vi "數位濾波版V2.vi"() -> ()   [LabVIEW 2010]
uses:
  <vilib>/Analysis/3filter.llb/Filter Passband Type.ctl
  <vilib>/DAQmx/read.llb/DAQmx Read (Analog DBL 1Chan 1Samp).vi
  <vilib>/DAQmx/write.llb/DAQmx Write (Analog DBL 1Chan 1Samp).vi
  <vilib>/DAQmx/create/channels.llb/DAQmx Create Channel (AI-Voltage-Basic).vi
  <vilib>/DAQmx/configure/timing.llb/DAQmx Timing (Sample Clock).vi
  <vilib>/DAQmx/create/channels.llb/DAQmx Create Channel (AO-Voltage-Basic).vi
  <vilib>/daqmx/miscellaneous.llb/DAQmx Fill In Error Info.vi
  <vilib>/Analysis/3filter.llb/Butterworth Filter (DBL).vi
  <vilib>/Analysis/NI_AALBase.lvlib
panel:
  in  "濾波?":bool
  in  "low cutoff freq: fl":dbl=200.0 format="%0.4f"
  out "理想迴圈時間":dbl
  out "延遲警告":bool
  in  "濾波階數":i32=6
  out "當下DC值":dbl
  in  "DAQ input":tag
  in  "DAQ output":tag
  in  "平均數":i32=1
  in  "ÂoDC«á©ñ¤j":dbl=1.0
  in  "Kp":dbl=1.0
  out "當下誤差":dbl=0.1 format="%#_13g"
  out "message":string=" INSTRUCTIONS:\r\rNormal Use:  When using subVIs that incorporate the error in/error out (or error I/O) structure, place this handler where you want to inform the user of an error, typically at the end of the I/O data path, as the last action of the program.  If the error in error? is ERROR, the handler creates a message describing the error and its source.  If the type of dialog = 1 (default), the message is displayed to the user, who can only acknowedge it.  If the type = 2, the user can acknowledge the message or abort execution; aborting a program with active I/O is not recommended.  If the type = 0, no message is displayed; this is used to process the error programmatically, and the error out cluster elements are wired to individual terminals for that reason.  \r\rOther Use:\n\r\nlocal testing.  To test the error code of a subVI or function that does not have the error I/O structure, you can wire its error code and a source string to the local error code and error source inputs.  If error in error? indicates no error and error code is not equal to 0, the local code and source are substituted for the error in values, and error? is set TRUE (ERROR)."
  out "while平均運行時間":dbl
  in  "取樣頻率":dbl=9000.0 min=1.0 max=20000.0 step=1.0
  in  "stop":bool
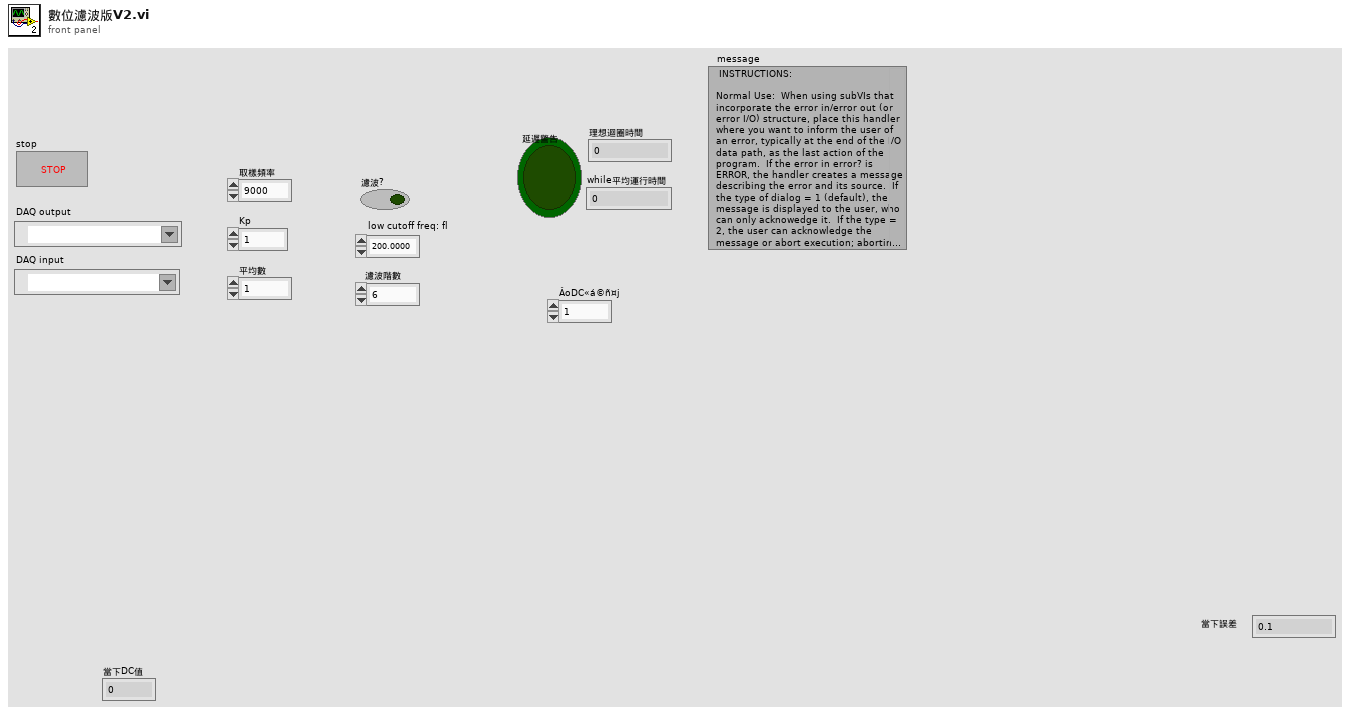
[diagram p1: front panel]
types:
  T1 = typedef "NI_AALBase.lvlib/Filter Passband Type.ctl" = enum32{"Lowpass", "Highpass", "Bandpass", "Bandstop"}
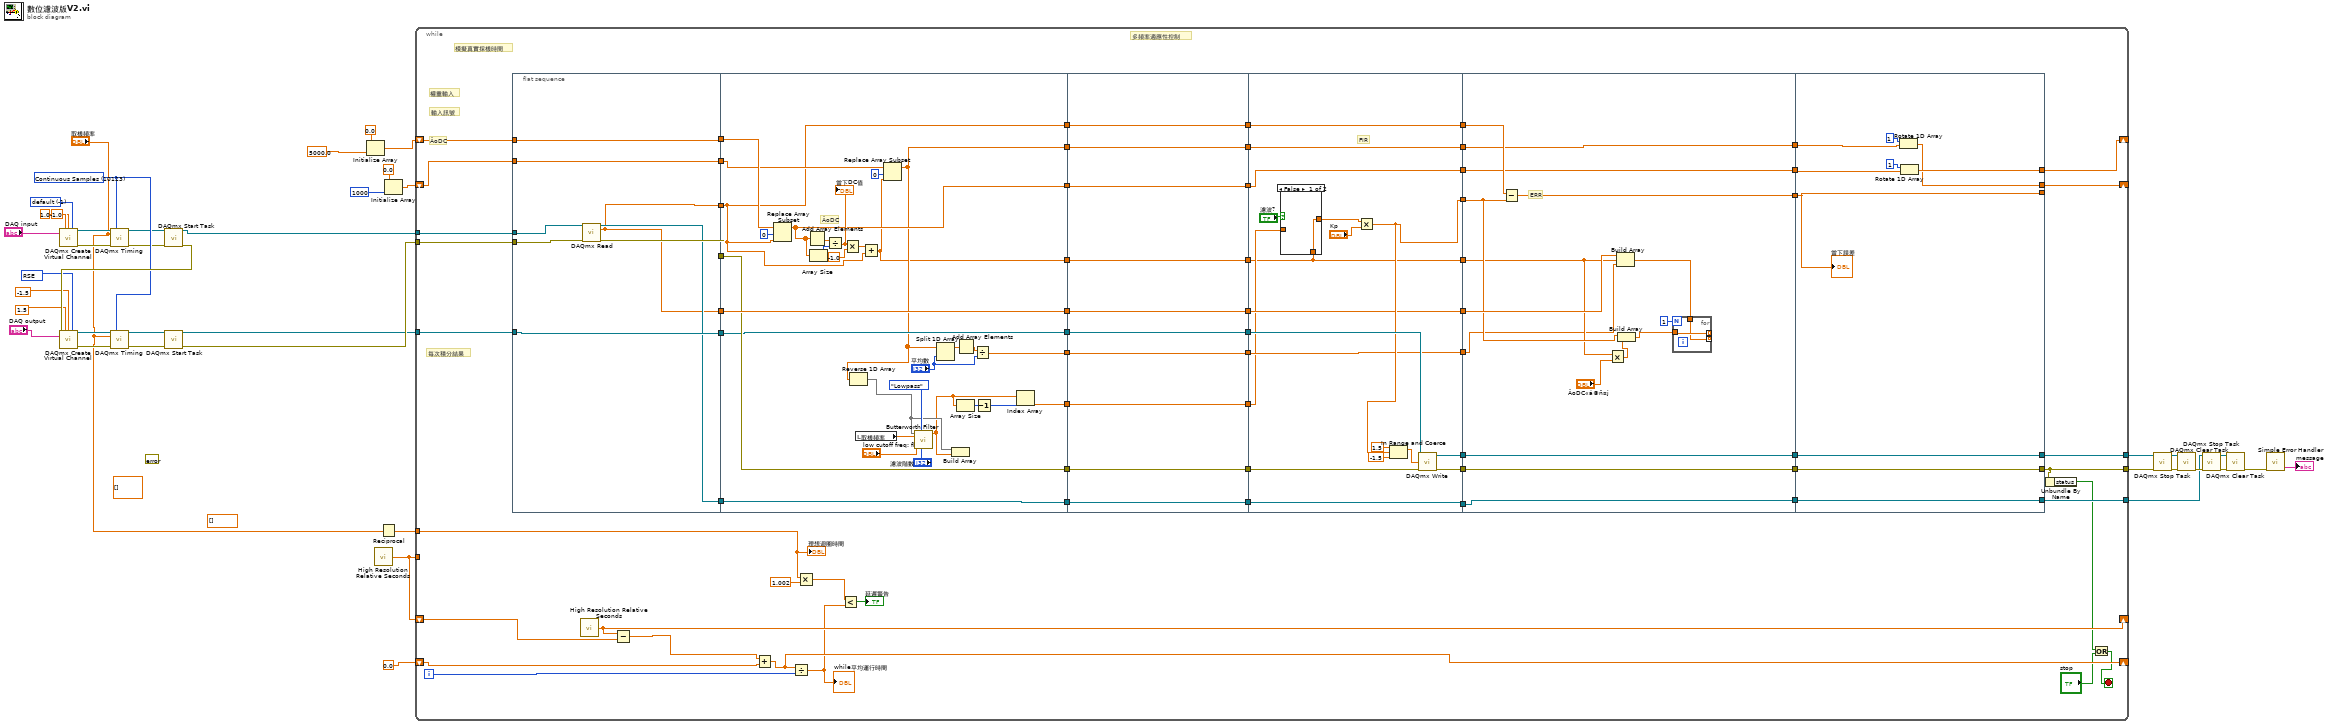
[diagram p0: block diagram]
diagram:
  w34 = 10123 items=["Finite Samples"=10178, "Continuous Samples"=10123, "Hardware Timed Single Point"=12522] ("sample mode")
  w31 = 10083 items=["Default"=-1, "RSE"=10083, "Differential"=10106, "Pseudodifferential"=12529] ("output terminal configuration")
  w30 = -1 items=["default"=-1, "RSE"=10083, "NRSE"=10078, "Differential"=10106, "Pseudodifferential"=12529] ("input terminal configuration")
  (unwired) dbl[] [] ("History Data")
  (unwired) dbl[][] [] ("History Data")
  (unwired) errorcluster {"status"=FALSE, "code"=0, "source"=""} ("error constant")
  n1 = call-poly <vilib>:"DAQmx Create Virtual Channel.vi"("maximum value"=1.0, "minimum value"=-1.0, "input terminal configuration"=w30, "physical channels"="DAQ input") -> ("task out"=w22:refnum<k21>, "error out"=w25:errorcluster)  [unwired: 10 in]
  n2 = call-poly <vilib>:"DAQmx Timing.vi"("task/channels in"=w22, "sample mode"=w34, "rate"="取樣頻率", "error in"=w25) -> ("task out"=w23:refnum<k21>, "error out"=w24:errorcluster)  [unwired: 10 in]
  n3 = call <vilib>:"DAQmx Start Task.vi"("task/channels in"=w23, "error in"=w24) -> ("task out"=w21:refnum<k21>, "error out"=w37:errorcluster)  [unwired: 12 in]
  n4 = call-poly <vilib>:"DAQmx Create Virtual Channel.vi"("maximum value"=1.5, "minimum value"=-1.5, "output terminal configuration"=w31, "physical channels"="DAQ output", "error in"=w37) -> ("task out"=w29:refnum<k21>, "error out"=w26:errorcluster)  [unwired: 9 in]
  n5 = call-poly <vilib>:"DAQmx Timing.vi"("task/channels in"=w29, "sample mode"=w34, "rate"="取樣頻率", "error in"=w26) -> ("task out"=w28:refnum<k21>, "error out"=w27:errorcluster)  [unwired: 10 in]
  n6 = call <vilib>:"DAQmx Start Task.vi"("task/channels in"=w28, "error in"=w27) -> ("task out"=w19:refnum<k21>, "error out"=w20:errorcluster)  [unwired: 12 in]
  n7 = Initialize Array(0.0 ("element"), 5000.0 ("y")) -> (w7:dbl[])
  n8 = call <vilib>:"High Resolution Relative Seconds.vi"() -> ("relative seconds"=w41:dbl)
  n9 = Reciprocal(x="取樣頻率") -> (1/x=w1:dbl)
  n10 = Initialize Array(0.0 ("element"), 1000 ("dimension size")) -> (w5:dbl[])
  n11 = while {
    tunnel: w41 -> [_]
    shift-right: [w103] -> _
    shift-left: w41 -> [w102]
    shift-right: [w104] -> _
    shift-left: 0.0 -> [w106]
    shift-right: [w94] -> _
    shift-left: w7 -> [w96]
    tunnel: w21 -> [w90]
    tunnel: w20 -> [w89]
    tunnel: w19 -> [w88]
    tunnel: [w84] -> w13
    tunnel: [w75] -> w12
    tunnel: [w78] -> w11
    shift-right: [w50] -> _
    shift-left: w5 -> [w55]
    tunnel: w1 -> [w46]
    i -> [w105]
    stop <- w77 stop-if-true
    # "每次積分結果"
    # "權重輸入"
    # "輸入訊號"
    # "ÂoDC"
    # "模擬真實採樣時間"
    # "多頻率適應性控制"
    n12 = flat-sequence {
      tunnel: [w109] -> w108
      tunnel: [w109] -> w100
      tunnel: [w113] -> w99
      tunnel: w96 -> [w116]
      tunnel: [w116] -> w95
      tunnel: w90 -> [w115]
      tunnel: w89 -> [w114]
      tunnel: w88 -> [w112]
      tunnel: [w112] -> w87
      tunnel: [w111] -> w81
      tunnel: [w110] -> w56
      tunnel: w55 -> [w110]
      tunnel: w108 -> [w118]
      tunnel: [w145] -> w72
      tunnel: [w146] -> w70
      tunnel: w100 -> [w146]
      tunnel: w99 -> [w145]
      tunnel: [w118] -> w68
      tunnel: w95 -> [w143]
      tunnel: [w132] -> w66
      tunnel: [w117] -> w64
      tunnel: [w133] -> w62
      tunnel: [w135] -> w60
      tunnel: w87 -> [w135]
      tunnel: [w134] -> w58
      tunnel: w81 -> [w134]
      tunnel: w56 -> [w129]
      tunnel: [w125] -> w51
      tunnel: [w126] -> w49
      tunnel: w72 -> [w156]
      tunnel: [w156] -> w71
      tunnel: w70 -> [w155]
      tunnel: [w155] -> w69
      tunnel: w68 -> [w154]
      tunnel: [w154] -> w67
      tunnel: w66 -> [w153]
      tunnel: [w153] -> w65
      tunnel: w64 -> [w152]
      tunnel: [w152] -> w63
      tunnel: w62 -> [w151]
      tunnel: [w151] -> w61
      tunnel: w60 -> [w150]
      tunnel: [w150] -> w59
      tunnel: w58 -> [w149]
      tunnel: [w149] -> w57
      tunnel: [w148] -> w52
      tunnel: w51 -> [w148]
      tunnel: w49 -> [w147]
      tunnel: [w147] -> w48
      tunnel: w71 -> [w171]
      tunnel: [w161] -> w101
      tunnel: w69 -> [w161]
      tunnel: [w174] -> w98
      tunnel: w67 -> [w174]
      tunnel: [w163] -> w97
      tunnel: [w173] -> w92
      tunnel: w65 -> [w173]
      tunnel: w63 -> [w157]
      tunnel: [w157] -> w91
      tunnel: w61 -> [w162]
      tunnel: w59 -> [w172]
      tunnel: [w170] -> w85
      tunnel: [w169] -> w83
      tunnel: w57 -> [w168]
      tunnel: [w168] -> w80
      tunnel: [w162] -> w73
      tunnel: [w164] -> w53
      tunnel: w52 -> [w164]
      tunnel: w48 -> [w159]
      tunnel: [w192] -> w107
      tunnel: w101 -> [w190]
      tunnel: w98 -> [w191]
      tunnel: w97 -> [w188]
      tunnel: [w180] -> w93
      tunnel: w92 -> [w180]
      tunnel: w91 -> [w187]
      tunnel: [w184] -> w86
      tunnel: w85 -> [w184]
      tunnel: w83 -> [w183]
      tunnel: [w183] -> w82
      tunnel: w80 -> [w182]
      tunnel: [w182] -> w79
      tunnel: w73 -> [w181]
      tunnel: [w178] -> w54
      tunnel: w53 -> [w178]
      tunnel: w107 -> [w205]
      tunnel: [w205] -> _
      tunnel: [w203] -> w94
      tunnel: w93 -> [w202]
      tunnel: w86 -> [w201]
      tunnel: [w201] -> w84
      tunnel: [w200] -> w75
      tunnel: w82 -> [w200]
      tunnel: w79 -> [w199]
      tunnel: [w199] -> w78
      tunnel: w54 -> [w197]
      tunnel: [w196] -> w50
      frame #0 {
        n13 = call-poly <vilib>:"DAQmx Read.vi"("task/channels in"=w115, "error in"=w114) -> ("task out"=w111:refnum<k21>, "data"=w109:dbl, "error out"=w113:errorcluster)  [unwired: 11 in]
      }
      frame #1 {
        # "ÂoDC"
        n14 = Replace Array Subset(array=w143, new element=w118, index=0) -> (w132:dbl[])
        n15 = Add Array Elements(numeric array=w132) -> (sum=w142:dbl)
        n16 = Array Size(array=w132) -> (size(s)=w141:i32)
        n17 = Divide(x=w142, y=w141) -> (x/y=w140:dbl)
        "當下DC值" <- w140
        n18 = Multiply(x=w140, y=-1.0) -> (x*y=w138:dbl)
        n19 = local read "取樣頻率"() -> (w128:dbl)
        n20 = Add(x=w138, y=w118) -> (x+y=w117:dbl)
        n21 = Replace Array Subset(array=w129, new element=w117, index=0) -> (w125:dbl[])
        n22 = Reverse 1D Array(array=w125) -> (reversed array=w124:dbl[])
        n23 = call-poly <vilib>:"Butterworth Filter.vi"("order"="濾波階數", "filter type"=Filter_Passband_Type."Lowpass", "low cutoff freq: fl"="low cutoff freq: fl", "sampling freq: fs"=w128, "X"=w124) -> ("Filtered X"=w123:dbl[])  [unwired: 3 in, 1 out]
        n24 = Split 1D Array(array=w125, index="平均數") -> (first subarray=w131:dbl[])  [unwired: 1 out]
        n25 = Build Array(w124, w123) -> ()  [unwired: 1 out]
        n26 = Array Size(array=w123) -> (size(s)=w122:i32)
        n27 = Add Array Elements(numeric array=w131) -> (sum=w137:dbl)
        n28 = Divide(x=w137, y="平均數") -> (x/y=w133:dbl)
        n29 = Decrement(x=w122) -> (x-1=w121:i32)
        n30 = Index Array(array=w123, index=w121) -> (element=w126:dbl)
      }
      frame #2 {
      }
      frame #3 {
        # "FIR"
        n31 = case shown="False" "濾波?" {
          tunnel: w159 -> [_ w177]
          tunnel: [w176 w177] -> w158
          tunnel: w157 -> [w176 _]
          frame False {
          }
          frame True {
          }
        }
        n32 = Multiply(x=w158, y="Kp") -> (x*y=w163:dbl)
        n33 = In Range and Coerce(upper limit=1.5, x=w163, lower limit=-1.5) -> (coerced(x)=w167:dbl)  [unwired: 1 out]
        n34 = call-poly <vilib>:"DAQmx Write.vi"("task/channels in"=w172, "data"=w167, "error in"=w171) -> ("task out"=w170:refnum<k21>, "error out"=w169:errorcluster)  [unwired: 10 in, 1 out]
      }
      frame #4 {
        # "ERR"
        n35 = Subtract(x=w191, y=w188) -> (x-y=w192:dbl)
        n36 = Multiply(x=w187, y="ÂoDC«á©ñ¤j") -> (x*y=w185:dbl)
        n37 = Build Array(w190, w187, w181) -> (w189:dbl[])
        n38 = Build Array(w188, w185) -> (w179:dbl[])
        n39 = for {
          N: 1 -> [_]
          tunnel: [w195] -> _ mode=indexing
          tunnel: w179 -> [w195]
          tunnel: [w194] -> _ mode=indexing
          tunnel: w189 -> [w194]
        }
      }
      frame #5 {
        n40 = Rotate 1D Array(1:w197, 2:1 ("n")) -> (0:w196:dbl[])
        n41 = Rotate 1D Array(1:w202, 2:1 ("n")) -> (0:w203:dbl[])
        "當下誤差" <- w205
      }
    }
    n42 = call <vilib>:"High Resolution Relative Seconds.vi"() -> ("relative seconds"=w103:dbl)
    n43 = Subtract(x=w103, y=w102) -> (x-y=w47:dbl)
    n44 = Add(x=w47, y=w106) -> (x+y=w104:dbl)
    n45 = Divide(x=w104, y=w105) -> (x/y=w43:dbl)
    "while平均運行時間" <- w43
    n46 = Multiply(x=w46, y=1.002) -> (x*y=w44:dbl)
    n47 = Less?(x=w44, y=w43) -> (x < y?=→"延遲警告":bool)
    n48 = Unbundle By Name(w75) -> ("status"=w74:bool)
    n49 = Or(x=w74, y="stop") -> (x .or. y?=w77:bool)
    "理想迴圈時間" <- w46
  }
  n50 = call <vilib>:"DAQmx Stop Task.vi"("task/channels in"=w13, "error in"=w12) -> ("task out"=w14:refnum<k21>, "error out"=w15:errorcluster)  [unwired: 12 in]
  n51 = call <vilib>:"DAQmx Clear Task.vi"("task in"=w14, "error in"=w15) -> ("error out"=w18:errorcluster)  [unwired: 13 in]
  n52 = call <vilib>:"DAQmx Stop Task.vi"("task/channels in"=w11, "error in"=w18) -> ("task out"=w17:refnum<k21>, "error out"=w16:errorcluster)  [unwired: 12 in]
  n53 = call <vilib>:"DAQmx Clear Task.vi"("task in"=w17, "error in"=w16) -> ("error out"=w10:errorcluster)  [unwired: 13 in]
  n54 = call <vilib>:"Simple Error Handler.vi"("error in (no error)"=w10) -> ("message"=→"message":string)  [unwired: 4 in, 4 out]
